vi "update freq in ui.vi"(8 "error in (no error)":errorcluster caption="에러 입력(에러 없음)", 10 "sampling rate":u32, 11 "Haptic IC 입력":refnum<class "Haptic IC.lvclass">) -> (0 "error out":errorcluster caption="에러 출력", 3 "Haptic IC 출력":refnum<class "Haptic IC.lvclass">)   [LabVIEW 2020, in "Haptic IC.lvclass"]
uses:
  Haptic IC.lvclass
  Haptic IC.lvclass/Haptic IC.ctl
  Accessors/Read freq ref.vi
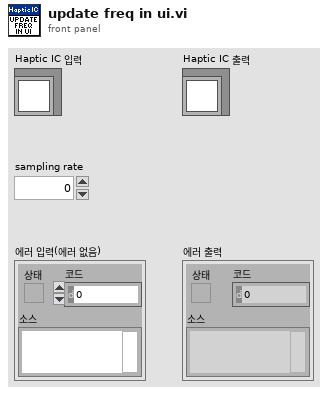
[diagram p1: front panel]
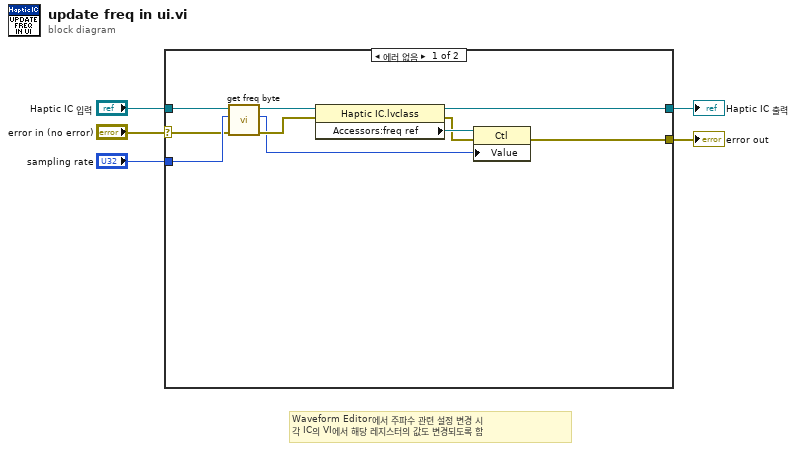
[diagram p0: block diagram]
diagram:
  # "Waveform Editor에서 주파수 관련 설정 변경 시\n각 IC의 VI에서 해당 레지스터의 값도 변경되도록 함"
  n1 = case shown="에러 없음" "error in (no error)" {
    selector: "error in (no error)" -> [w7 w17]
    tunnel: [w6 w17] -> w4
    tunnel: [w14 w16] -> w2
    tunnel: "Haptic IC 입력" -> [w15 w16]
    tunnel: "sampling rate" -> [w9 _]
    frame No Error {
      n2 = call-dynamic "get freq byte.vi"("error in (no error)"=w7, "freq"=w9, "Haptic IC 입력"=w15) -> ("error out"=w10:errorcluster, "byte value"=w8:u8, "Haptic IC 출력"=w11:refnum<class "Haptic IC.lvclass">)  [unwired: 6 in]
      n3 = property class="Haptic IC.lvclass"(reference=w11, error in=w10) -> (reference out=w14:refnum<class "Haptic IC.lvclass">, error out=w12:errorcluster, "Accessors:freq ref"=w13:refnum<vi>)
      n4 = property class="Ctl"(reference=w13, error in=w12, "Value"=w8) -> (error out=w6:errorcluster)  [unwired: 1 out]
    }
    frame Error {
    }
  }
  "error out" <- w4
  "Haptic IC 출력" <- w2
